vi "Start-stop.vi"(8 "Error In":errorcluster, 9 "Motor index":u8, 10 "Go":bool, 11 "VISA resource in":refnum<visa-resource-name>) -> (0 "Error Out":errorcluster, 3 "VISA resource out":refnum<visa-resource-name>)   [LabVIEW 2014, in "Motor manager.lvlib"]
uses:
  Motor manager.lvlib
  Typedef/Commands.ctl
  Cmd to Byte Array (Sgl).vi
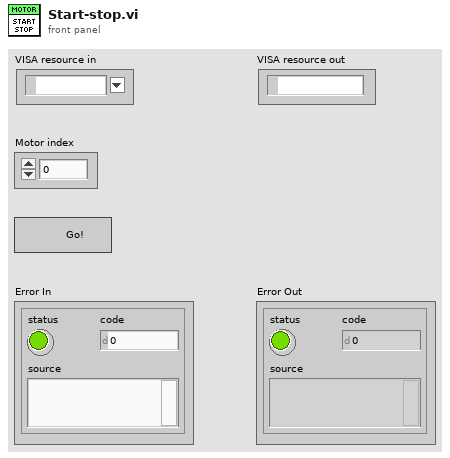
[diagram p1: front panel]
types:
  T1 = typedef "Motor manager.lvlib/Commands.ctl" = enum16{"None", "Set motor", "Set distance", "Set speed", "Set Move Type", "Set IM Idle Time", "Set N cycles", "Start", "Stop", "Stop and Release", "Set Home", "Find Home", "Move Forward", "Move Backward"}
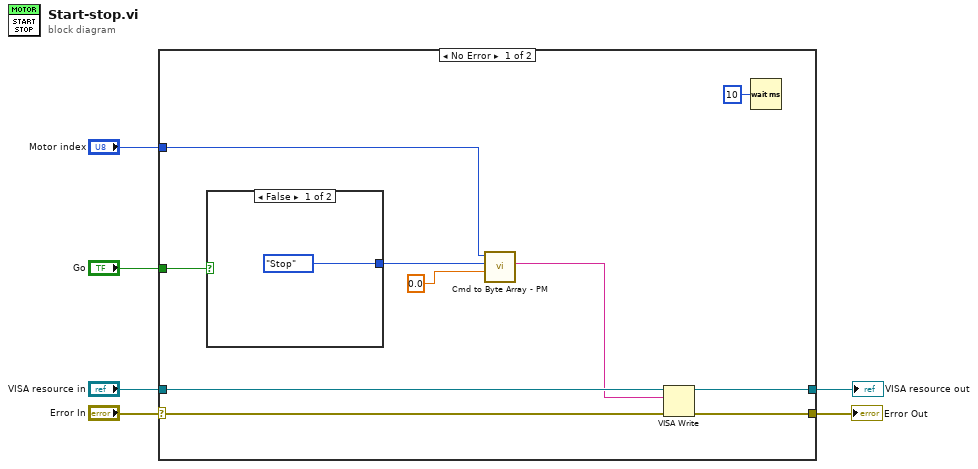
[diagram p0: block diagram]
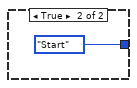
[diagram p2: hidden frame]
diagram:
  n1 = case shown="No Error" "Error In" {
    selector: "Error In" -> [w16 w20]
    tunnel: [w15 w20] -> w5
    tunnel: "VISA resource in" -> [w14 w19]
    tunnel: [w13 w19] -> w3
    tunnel: "Go" -> [w12 _]
    tunnel: "Motor index" -> [w8 _]
    frame No Error {
      n2 = case shown="False" w12 {
        tunnel: [Commands."Stop" ("Commands") Commands."Start" ("Commands")] -> w10
        frame False {
        }
        frame True {
        }
      }
      n3 = call-poly "Cmd to Byte Array - PM.vi"("Parameter"=sgl 0.0, "Commands"=w10, "Motor index"=w8) -> ("Byte string"=w11:string)  [unwired: 8 in]
      n4 = VISA Write(VISA resource name=w14, write buffer=w11, error in (no error)=w16) -> (VISA resource name out=w13:refnum<visa-resource-name>, error out=w15:errorcluster)  [unwired: 1 out]
      n5 = Wait (ms)(milliseconds to wait=u32 10) -> ()  [unwired: 1 out]
    }
    frame Error {
    }
  }
  "Error Out" <- w5
  "VISA resource out" <- w3
